vi "get_phase_duration.vi"(8 "error in (no error)":errorcluster, 11 "ScanModeMG091111IntrinsicImaging in":refnum<class "ImagingModeMG091111IntrinsicImaging.lvclass">) -> (0 "error out":errorcluster, 2 "phase duration":dbl[unit], 3 "ScanModeMG091111IntrinsicImaging out":refnum<class "ImagingModeMG091111IntrinsicImaging.lvclass">)   [LabVIEW 2010, in "ImagingModeMG091111IntrinsicImaging.lvclass"]
uses:
  ImagingModeMG091111IntrinsicImaging.lvclass
  ImagingModeMG091111IntrinsicImaging.lvclass/ImagingModeMG091111IntrinsicImaging.ctl
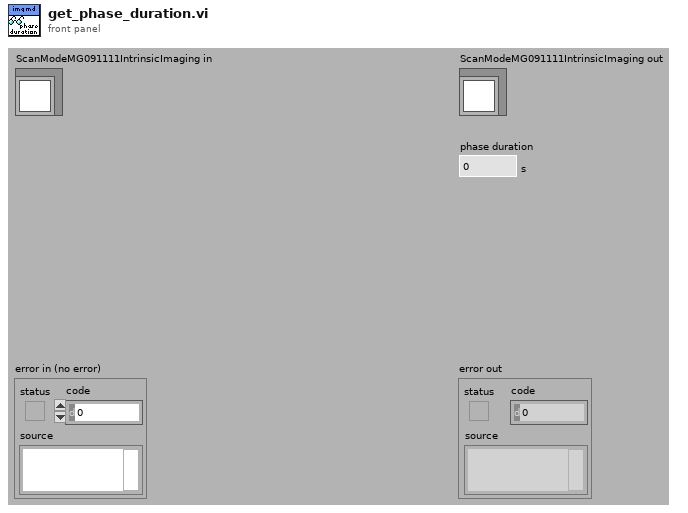
[diagram p1: front panel]
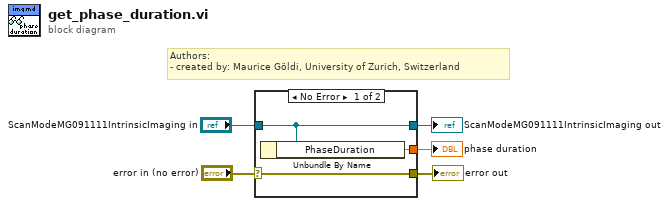
[diagram p0: block diagram]
diagram:
  # "Authors: \n- created by: Maurice Göldi, University of Zurich, Switzerland"
  n1 = case shown="No Error" "error in (no error)" {
    selector: "error in (no error)" -> [w8 w9]
    tunnel: [w8 w9] -> w4
    tunnel: [w7 w10] -> w2
    tunnel: "ScanModeMG091111IntrinsicImaging in" -> [w7 w10]
    tunnel: [w6 _] -> w1
    frame No Error {
      n2 = Unbundle By Name(w7) -> ("PhaseDuration"=w6:dbl[unit])
    }
    frame Error {
    }
  }
  "error out" <- w4
  "ScanModeMG091111IntrinsicImaging out" <- w2
  "phase duration" <- w1
